vi "FTW-Endpoint-Core-LibraryFilepath.vi"(8 "error in":errorcluster) -> (0 "error out":errorcluster, 1 "Library Version":string, 2 "Library Filepath":path)   [LabVIEW 2013, in "FTW-Actor.lvlib" / "FTW-Endpoint.lvclass"]
uses:
  FTW-Endpoint.lvclass
  FTW-Endpoint-Symbols.vi
  Core/FTWLib-nanomsg-Win64.vi
  Core/FTWLib-nanomsg-Win32.vi
  Core/FTWLib-nanomsg-LinuxRT.vi
panel:
  # "Inputs"
  # "Outputs"
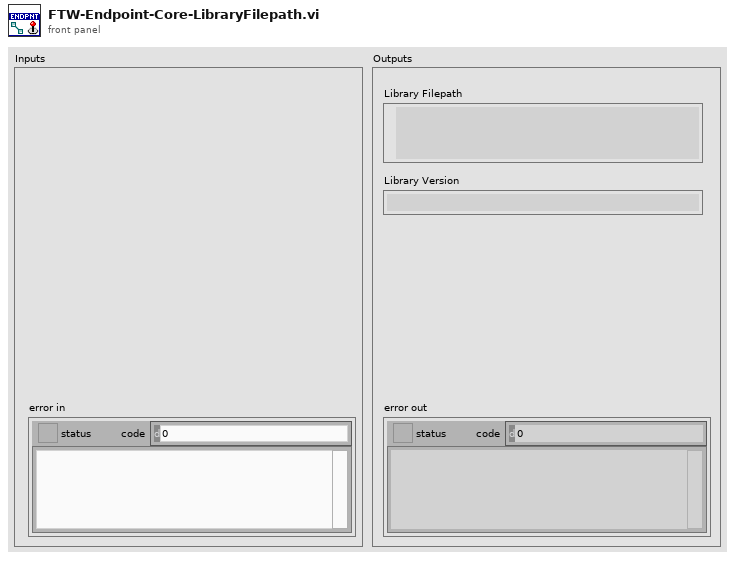
[diagram p1: front panel]
types:
  T1 = cluster{"Symbol Name":string, "Symbol Value":i32}
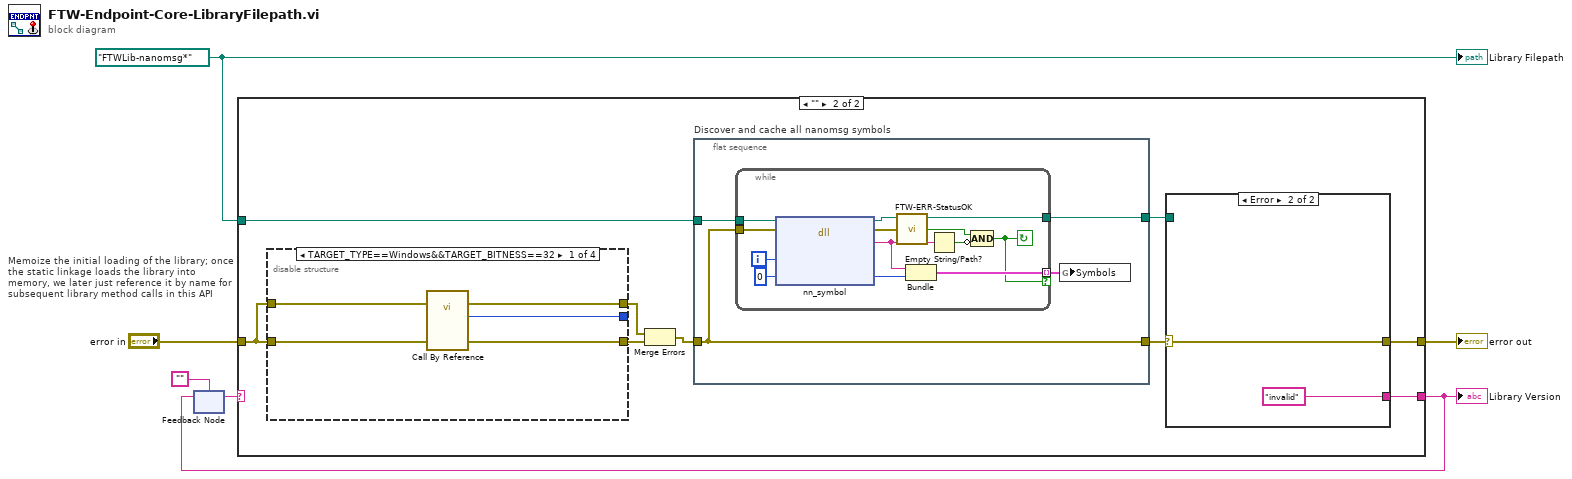
[diagram p0: block diagram]
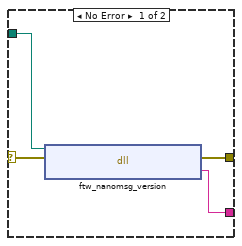
[diagram p3: hidden frame]
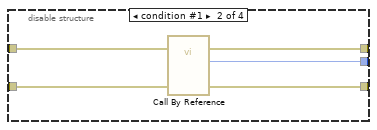
[diagram p4: hidden frame]
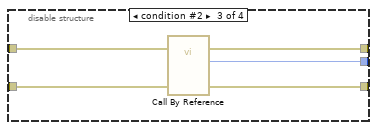
[diagram p5: hidden frame]
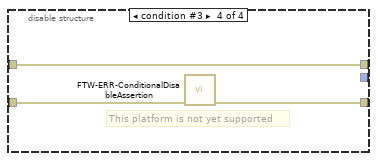
[diagram p6: hidden frame]
diagram:
  w1 = path "FTWLib-nanomsg*" ("nanomsg Library Filepath")
  n1 = feedback #1("") -> (w3:string)
  n2 = case "Memoize the initial loading of the library; once the static linkage loads the library into memory, we later just reference it by name for subsequent library method calls in this API" shown="\"\"" w3 {
    selector: w3 -> [w7 _]
    tunnel: "error in" -> [w8 w13]
    tunnel: [w7 w16] -> w4
    tunnel: [w8 w17] -> w5
    tunnel: w1 -> [_ w10]
    frame Default {
    }
    frame "" {
      n3 = disable-structure shown="TARGET_TYPE==Windows&&TARGET_BITNESS==32" {
        disable-tunnel: [w44 w46 w51 _] -> _
        disable-tunnel: [w43 w45 w50 w56] -> w14
        disable-tunnel: w13 -> [w41 w48 w53 w57]
        disable-tunnel: [w42 w47 w52 w55] -> w15
        disable-tunnel: w13 -> [w40 w49 w54 w55]
        frame condition #0 (active) {
          n4 = call-by-ref "?"(error in=w40, "error in"=w41) -> (error out=w42:errorcluster, "Integer Size"=w44:i32, 15:"error out"=w43:errorcluster)  [unwired: 14 in, 1 out]
        }
        frame condition #1 {
          n5 = call-by-ref "?"(error in=w49, "error in"=w48) -> (error out=w47:errorcluster, "Integer Size"=w46:i32, 15:"error out"=w45:errorcluster)  [unwired: 14 in, 1 out]
        }
        frame condition #2 {
          n6 = call-by-ref "?"(error in=w54, "error in"=w53) -> (error out=w52:errorcluster, "Integer Size"=w51:i32, 15:"error out"=w50:errorcluster)  [unwired: 14 in, 1 out]
        }
        frame condition #3 {
          # "This platform is not yet supported"
          n7 = call "FTW-ERR-ConditionalDisableAssertion.vi"("error in"=w57) -> ("error out"=w56:errorcluster)  [unwired: 14 in]
        }
      }
      n8 = Merge Errors(w15, w14) -> (w11:errorcluster)
      n9 = flat-sequence "Discover and cache all nanomsg symbols" {
        tunnel: [w21] -> w12
        tunnel: w11 -> [w21]
        tunnel: w10 -> [w19]
        tunnel: [w18] -> w9
        frame #0 {
          n10 = while {
            tunnel: w21 -> [w33]
            tunnel: [w30] -> w20 mode=indexing if=w25
            tunnel: w19 -> [w29]
            tunnel: [w22] -> w18
            i -> [w32]
            stop <- w25 continue-if-true
            n11 = dll-call lib="?" fn="nn_symbol"(path in=w29, error in=w33, "Symbol Index"=w32, "Symbol Value"=0) -> (path out=w22:path, error out=w24:errorcluster, "Symbol Name"=w28:string, "Symbol Value"=w31:i32)  [unwired: 2 in]
            n12 = call "FTW-ERR-StatusOK.vi"("error to check"=w24) -> ("Status OK?"=w27:bool)
            n13 = Bundle("Symbol Name"=w28, "Symbol Value"=w31) -> (w30:T1)  [unwired: 1 in]
            n14 = Empty String/Path?(string/path=w28) -> (empty?=w26:bool)
            n15 = Compound Arithmetic op=AND(w27, invert w26) -> (w25:bool)
          }
          n16 = global write "FTW-Endpoint-Symbols.vi" "Symbols"(w20) -> ()
        }
      }
      n17 = case shown="Error" w12 {
        selector: w12 -> [w37 w38]
        tunnel: [w34 w38] -> w17
        tunnel: [w35 "invalid" ("Version (minus Build)")] -> w16
        tunnel: w9 -> [w36 _]
        frame No Error {
          n18 = dll-call lib="?" fn="ftw_nanomsg_version"(path in=w36, error in=w37) -> (error out=w34:errorcluster, "nanomsg version"=w35:string)  [unwired: 1 in, 1 out]
        }
        frame Error {
        }
      }
    }
  }
  "error out" <- w5
  "Library Version" <- w4
  n19 = feedback-in #1(w4) -> ()
  "Library Filepath" <- w1
